vi "AllowEdgeStartCheck.vi"(0 "reference in":refnum<class "DqmhModuleDiagramGraph.lvclass">, 1 "EdgeStartNode":refnum<class "AbstractNode.lvclass">, 2 "GraphButton":u32, 5 "error in (no error)":errorcluster) -> (14 "reference out":refnum<class "DqmhModuleDiagramGraph.lvclass">, 16 "Allowed":bool, 19 "error out":errorcluster)   [LabVIEW 2020, in "DqmhModuleDiagramGraph.lvclass"]
uses:
  <resource>/Framework/Providers/Open_GDS/UML/DqmhModuleDiagramGraph_class/DqmhModuleDiagramGraph.lvclass
  <resource>/Framework/Providers/Open_GDS/UML/AbstractNode_class/AbstractNode.lvclass
  <resource>/Framework/Providers/Open_GDS/UML/Graph_class/ToolbarButtonType.ctl
  <resource>/Framework/Providers/Open_GDS/UML/UMLEditor/UMLEditor tooltype.ctl
  <resource>/Framework/Providers/Open_GDS/UML/Graph_class/Graph.lvclass
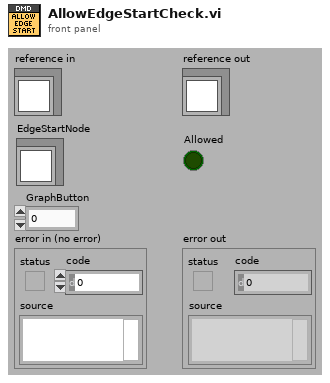
[diagram p1: front panel]
types:
  T1 = typedef "Graph.lvclass/ToolbarButtonType.ctl" = cluster{"Text":string, "Type":T2}
  T2 = typedef "UMLEditor tooltype.ctl" = enum16{"None", "Node", "Edge"}
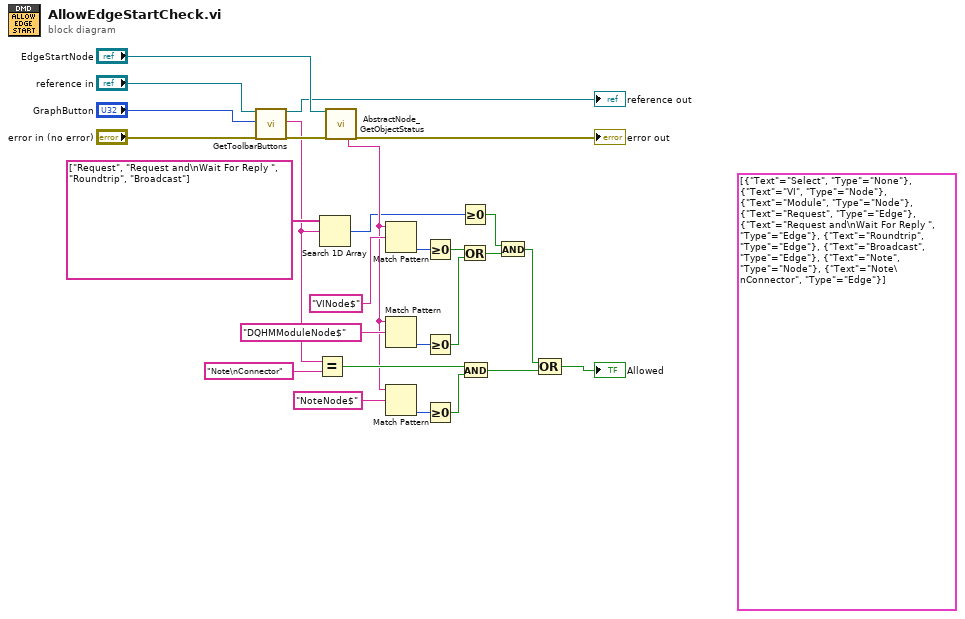
[diagram p0: block diagram]
diagram:
  (unwired) T1[] [{"Text"="Select", "Type"=enum."None"}, {"Text"="VI", "Type"=enum."Node"}, {"Text"="Module", "Type"=enum."Node"}, {"Text"="Request", "Type"=enum."Edge"}, {"Text"="Request and\nWait For Reply ", "Type"=enum."Edge"}, {"Text"="Roundtrip", "Type"=enum."Edge"}, {"Text"="Broadcast", "Type"=enum."Edge"}, {"Text"="Note", "Type"=enum."Node"}, {"Text"="Note\nConnector", "Type"=enum."Edge"}] ("ToolbarButtons")
  n1 = call-dynamic "GetToolbarButtons.vi"("reference in"="reference in", "GraphButton"="GraphButton", "error in (no error)"="error in (no error)") -> ("reference out"=→"reference out":refnum<class "DqmhModuleDiagramGraph.lvclass">, "Text"=w3:string, "error out"=w20:errorcluster)  [unwired: 12 in, 2 out]
  n2 = Equal?(x=w3, y="Note\nConnector" ("Text")) -> (x = y?=w10:bool)
  n3 = Search 1D Array(1D array=string[] ["Request", "Request and\nWait For Reply ", "Roundtrip", "Broadcast"], element=w3) -> (index of element=w2:i32)  [unwired: 1 in]
  n4 = call <resource>:"AbstractNode_GetObjectStatus.vi"("reference in"="EdgeStartNode", "error in (no error)"=w20) -> ("Class name"=w6:string, "error out"=→"error out":errorcluster)  [unwired: 16 out]
  n5 = Match Pattern(string=w6, regular expression="VINode$") -> (offset past match=w15:i32)  [unwired: 4 out]
  n6 = Match Pattern(string=w6, regular expression="DQHMModuleNode$") -> (offset past match=w14:i32)  [unwired: 4 out]
  n7 = Match Pattern(string=w6, regular expression="NoteNode$") -> (offset past match=w16:i32)  [unwired: 4 out]
  n8 = Greater Or Equal To 0?(x=w15) -> (x >= 0?=w13:bool)
  n9 = Greater Or Equal To 0?(x=w14) -> (x >= 0?=w12:bool)
  n10 = Greater Or Equal To 0?(x=w16) -> (x >= 0?=w9:bool)
  n11 = Greater Or Equal To 0?(x=w2) -> (x >= 0?=w1:bool)
  n12 = Or(x=w13, y=w12) -> (x .or. y?=w11:bool)
  n13 = And(x=w10, y=w9) -> (x .and. y?=w7:bool)
  n14 = And(x=w1, y=w11) -> (x .and. y?=w8:bool)
  n15 = Compound Arithmetic op=OR(w8, w7) -> (→"Allowed":bool)
